vi "Perform Checks.vi"(4 "Owner Path (if applicable)":path, 6 "User VI Owner Status":T1, 8 "error in":errorcluster, 9 "New Filename":string, 10 "Selected Template VI or CTL name (including file extension)":string, 11 "Destination Folder":path) -> (0 "error out":errorcluster, 2 "Validated Filename of VI or CTL to be created (including extension)":string, 3 "Filepath of VI or CTL to be created":path)   [LabVIEW 2022 SP3]
doc: "Performs a few sanity checks in order to ensure that everything is ok before attempting to create a new VI based on these inputs. In other words, performs input validation.\n\nSanity checks:\n1. Destination folder exists\n2. Destination folder does not already contain a file with the same name and extension as is about to be created\n3. Selected Template VI or CTL exists\n4. Owner Library or Class exists (if applicable, meaning if the User VI was owned by a library or class)\n\nReturns a meaningful, informative error if any of the sanity checks failed."
uses:
  Owner Status (enum).ctl
  <vilib>/Utility/error.llb/Trim Whitespace One-Sided.vi
panel:
  # "Development\ncontrols/indicators useful for development and testing, but which are not outputs of the VI"
  # "Input\nInputs to the VI"
  # "Output\nOutputs of the VI"
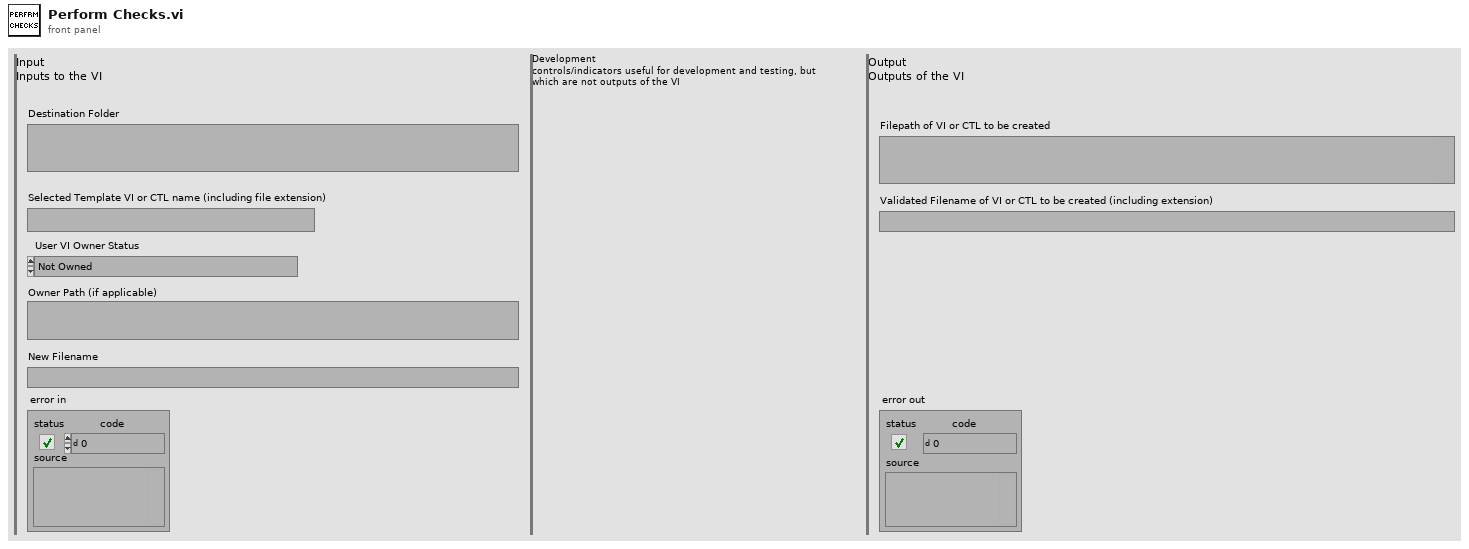
[diagram p1: front panel]
types:
  T1 = typedef "Owner Status (enum).ctl" = enum16{"Not Owned", "Owned by Library (lvlib)", "Owned by Class (lvclass)"}
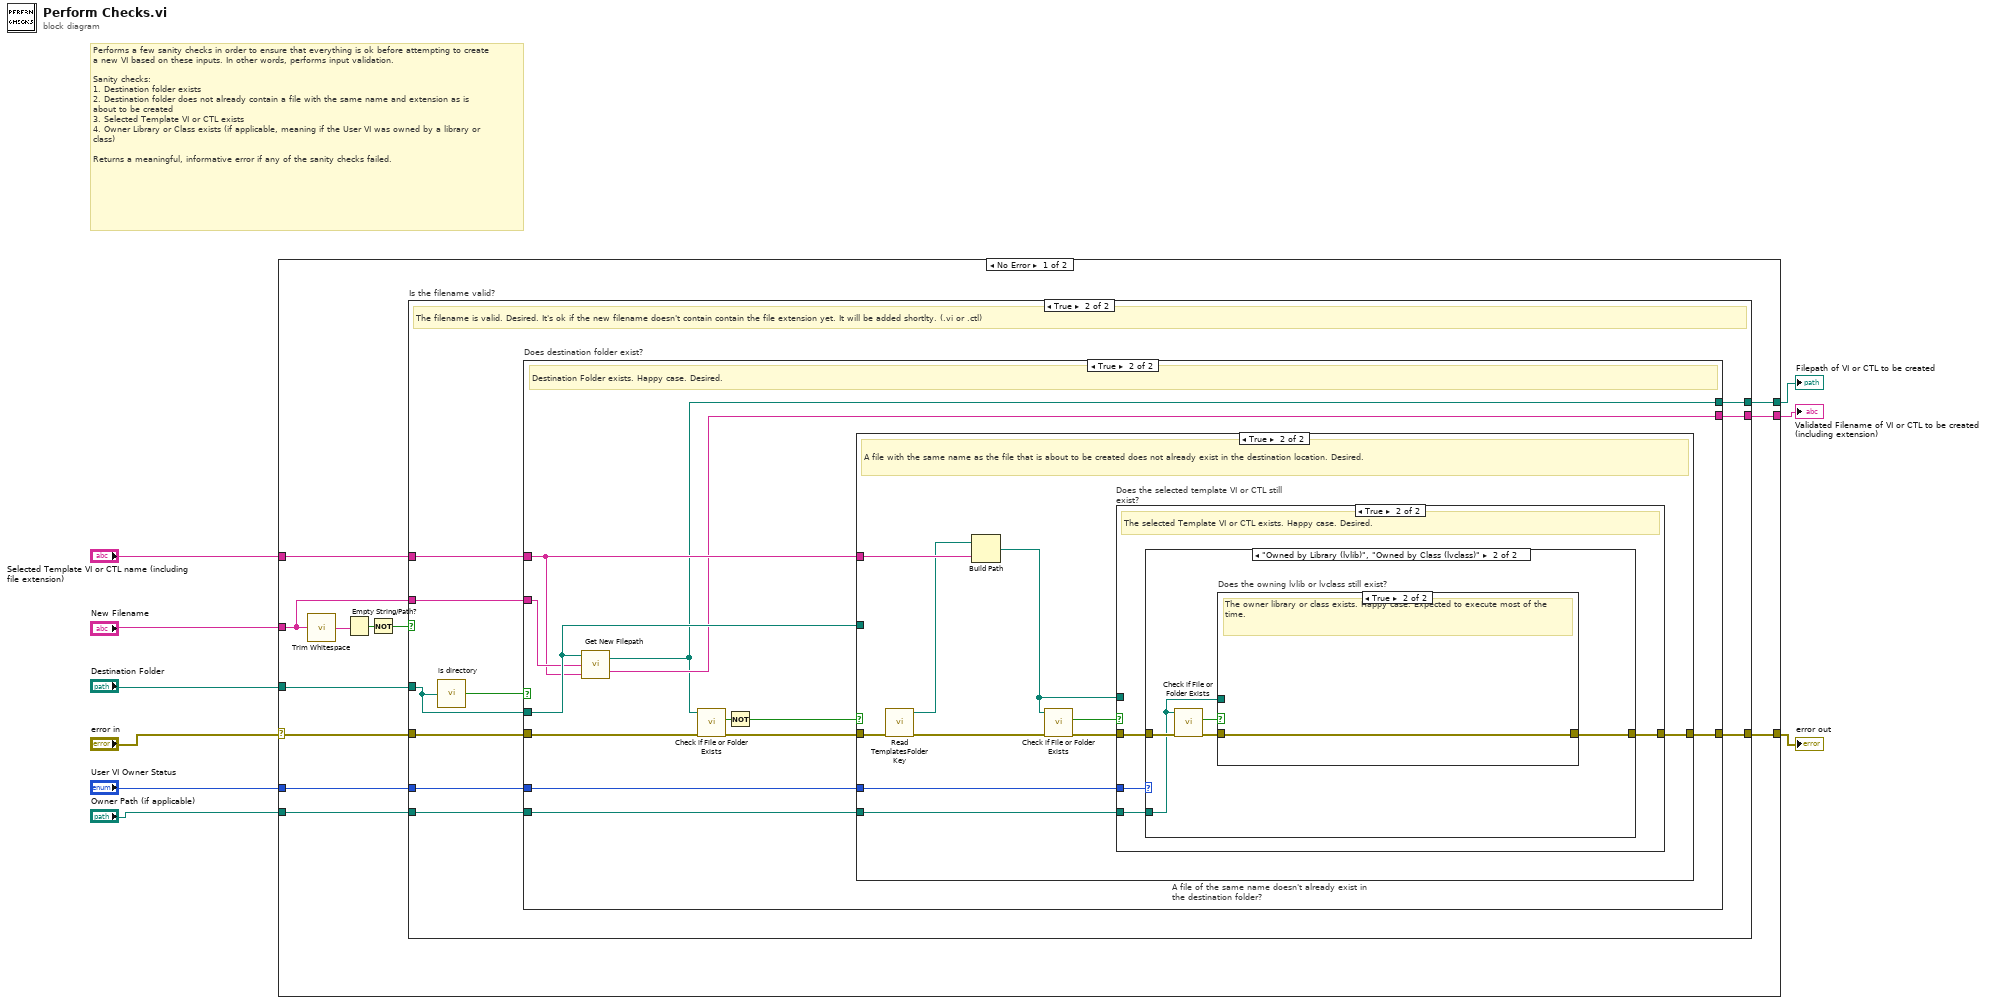
[diagram p0: block diagram]
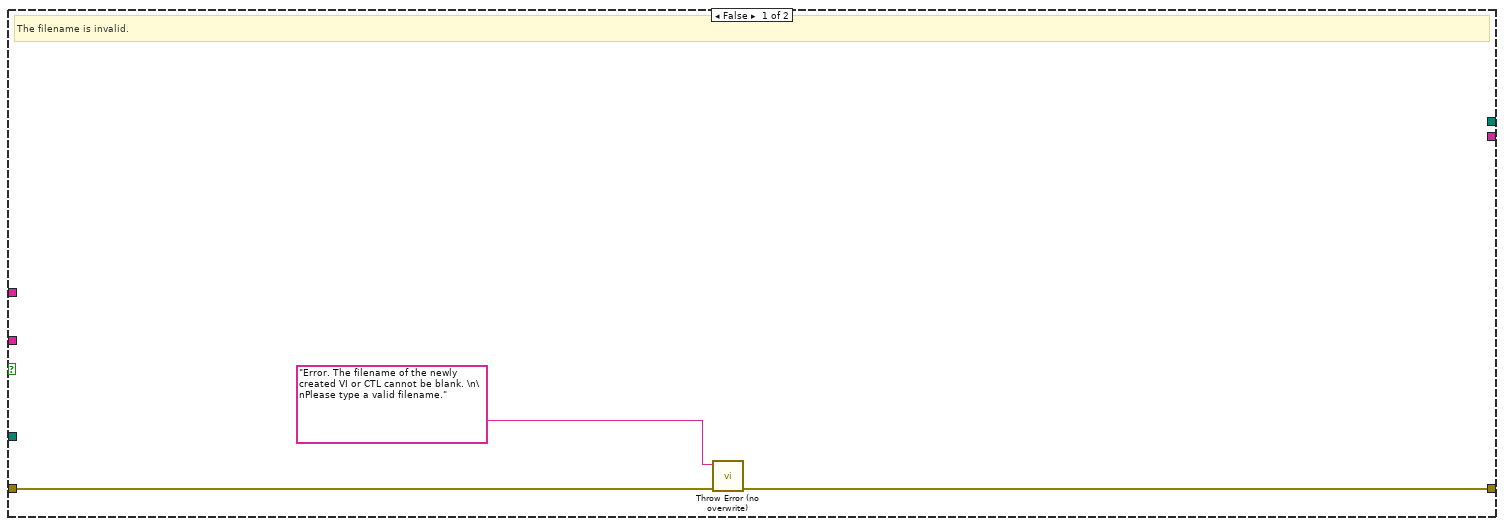
[diagram p2: hidden frame]
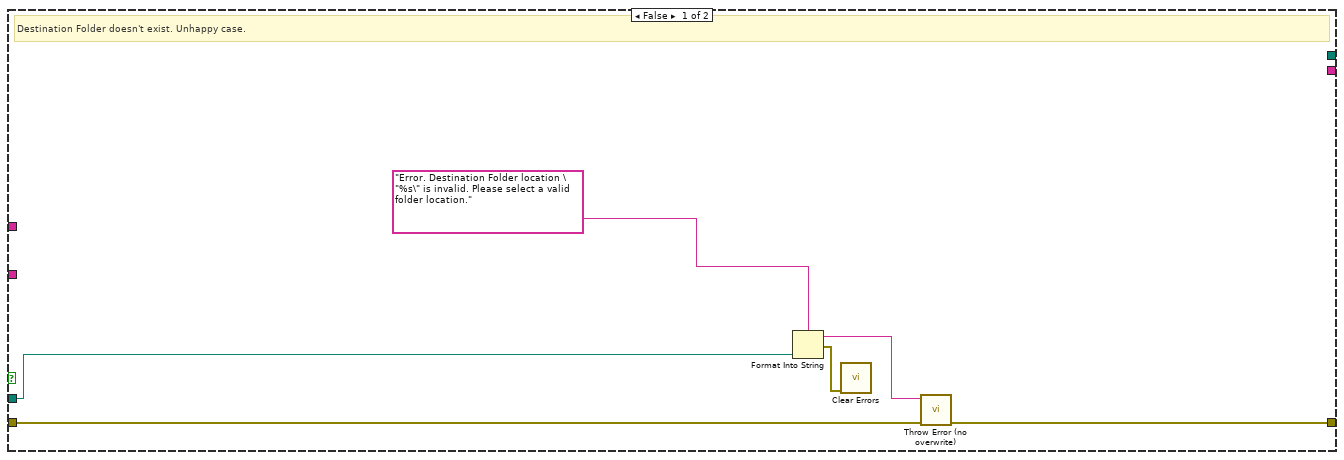
[diagram p3: hidden frame]
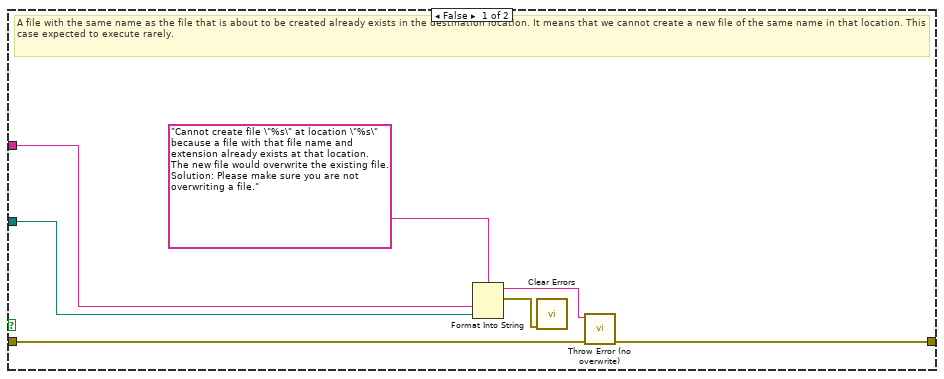
[diagram p4: hidden frame]
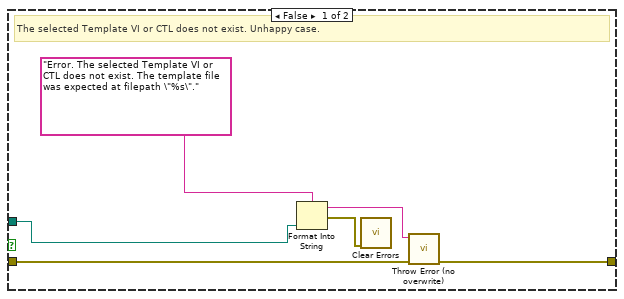
[diagram p5: hidden frame]
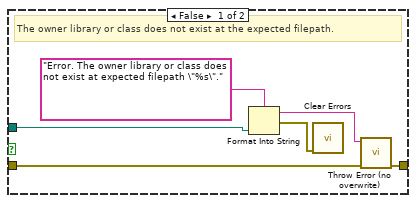
[diagram p7: hidden frame]
diagram:
  # "Performs a few sanity checks in order to ensure that everything is ok before attempting to create a new VI based on these inputs. In other words, performs input validation.\n\nSanity checks:\n1. Destination folder exists\n2. Destination folder does not already contain a file with the same name and extension as is about to be created\n3. Selected Template VI or CTL exists\n4. Owner Library or Class exists (if applicable, meaning if the User VI was owned by a library or class)\n\nReturns a meaningful, informative error if any of the sanity checks failed."
  n1 = case shown="No Error" "error in" {
    selector: "error in" -> [w21 w93]
    tunnel: [w20 w93] -> w8
    tunnel: "Destination Folder" -> [w16 _]
    tunnel: "Selected Template VI or CTL name (including file extension)" -> [w19 _]
    tunnel: "User VI Owner Status" -> [w18 _]
    tunnel: "Owner Path (if applicable)" -> [w17 _]
    tunnel: "New Filename" -> [w12 _]
    tunnel: [w11 _] -> w2
    tunnel: [w10 _] -> w1
    frame No Error {
      n2 = call <vilib>:"Trim Whitespace.vi"("string"=w12) -> ("trimmed string"=w14:string)  [unwired: 1 in]
      n3 = Empty String/Path?(string/path=w14) -> (empty?=w15:bool)
      n4 = Not(x=w15) -> (.not. x?=w13:bool)
      n5 = case "Is the filename valid?" shown="True" w13 {
        tunnel: w21 -> [w23 w34]
        tunnel: [w22 w33] -> w20
        tunnel: w19 -> [_ w32]
        tunnel: w18 -> [_ w31]
        tunnel: w17 -> [_ w30]
        tunnel: w16 -> [_ w29]
        tunnel: w12 -> [_ w27]
        tunnel: [_ w26] -> w11
        tunnel: [_ w25] -> w10
        frame False {
          # "The filename is invalid."
          n6 = call "Throw Error (no overwrite).vi"("error in"=w23, "Error Message"="Error. The filename of the newly created VI or CTL cannot be blank. \n\nPlease type a valid filename.") -> ("error out"=w22:errorcluster)  [unwired: 9 in]
        }
        frame True {
          # "The filename is valid. Desired. It's ok if the new filename doesn't contain contain the file extension yet. It will be added shortlty. (.vi or .ctl)"
          n7 = call "is directory.vi"("Path"=w29) -> ("Does the path point to a directory (a folder)?"=w28:bool)
          n8 = case "Does destination folder exist?" shown="True" w28 {
            tunnel: w34 -> [w40 w48]
            tunnel: [w39 w52] -> w33
            tunnel: w29 -> [w36 w45]
            tunnel: w32 -> [_ w43]
            tunnel: w31 -> [_ w51]
            tunnel: w30 -> [_ w50]
            tunnel: w27 -> [_ w44]
            tunnel: [_ w42] -> w26
            tunnel: [_ w41] -> w25
            frame False {
              # "Destination Folder doesn't exist. Unhappy case."
              n9 = Format Into String(format string="Error. Destination Folder location \"%s\" is invalid. Please select a valid folder location.", w36) -> (resulting string=w35:string, error out=w37:errorcluster)  [unwired: 2 in]
              n10 = call <vilib>:"Clear Errors.vi"("error in (no error)"=w37) -> ()  [unwired: 5 in, 2 out]
              n11 = call "Throw Error (no overwrite).vi"("error in"=w40, "Error Message"=w35) -> ("error out"=w39:errorcluster)  [unwired: 9 in]
            }
            frame True {
              # "Destination Folder exists. Happy case. Desired."
              n12 = call "Get New Filepath.vi"("Selected Template VI or CTL name (including file extension)"=w43, "New Filename"=w44, "Destination Folder"=w45) -> ("Validated Filename of VI or CTL to be created (including extension)"=w42:string, "Filepath of VI or CTL to be created"=w41:path)
              n13 = call <vilib>:"Check if File or Folder Exists.vi"("error in (no error)"=w48, "path"=w41) -> ("error out"=w49:errorcluster, "file or folder exists?"=w47:bool)  [unwired: 7 in, 1 out]
              n14 = Not(x=w47) -> (.not. x?=w46:bool)
              n15 = case "A file of the same name doesn't already exist in the destination folder?" shown="True" w46 {
                tunnel: w43 -> [w54 w69]
                tunnel: w49 -> [w56 w62]
                tunnel: [w55 w65] -> w52
                tunnel: w51 -> [_ w64]
                tunnel: w50 -> [_ w63]
                tunnel: w45 -> [w53 _]
                frame False {
                  # "A file with the same name as the file that is about to be created already exists in the destination location. It means that we cannot create a new file of the same name in that location. This case expected to execute rarely."
                  n16 = Format Into String(format string="Cannot create file \"%s\" at location \"%s\" because a file with that file name and extension already exists at that location. The new file would overwrite the existing file. Solution: Please make sure you are not overwriting a file.", w54, w53) -> (resulting string=w57:string, error out=w58:errorcluster)  [unwired: 2 in]
                  n17 = call <vilib>:"Clear Errors.vi"("error in (no error)"=w58) -> ()  [unwired: 5 in, 2 out]
                  n18 = call "Throw Error (no overwrite).vi"("error in"=w56, "Error Message"=w57) -> ("error out"=w55:errorcluster)  [unwired: 9 in]
                }
                frame True {
                  # "A file with the same name as the file that is about to be created does not already exist in the destination location. Desired."
                  n19 = call "Read TemplatesFolder Key.vi"("Error In"=w62) -> ("Error Out"=w61:errorcluster, "Templates Folder Path"=w60:path)  [unwired: 9 in]
                  n20 = Build Path(base path=w60, name or relative path=w69) -> (appended path=w66:path)
                  n21 = call <vilib>:"Check if File or Folder Exists.vi"("error in (no error)"=w61, "path"=w66) -> ("error out"=w68:errorcluster, "file or folder exists?"=w67:bool)  [unwired: 7 in, 1 out]
                  n22 = case "Does the selected template VI or CTL still exist?" shown="True" w67 {
                    tunnel: w68 -> [w75 w79]
                    tunnel: w66 -> [w71 _]
                    tunnel: [w70 w78] -> w65
                    tunnel: w64 -> [_ w77]
                    tunnel: w63 -> [_ w76]
                    frame False {
                      # "The selected Template VI or CTL does not exist. Unhappy case."
                      n23 = Format Into String(format string="Error. The selected Template VI or CTL does not exist. The template file was expected at filepath \"%s\".", w71) -> (resulting string=w72:string, error out=w73:errorcluster)  [unwired: 2 in]
                      n24 = call <vilib>:"Clear Errors.vi"("error in (no error)"=w73) -> ()  [unwired: 5 in, 2 out]
                      n25 = call "Throw Error (no overwrite).vi"("error in"=w75, "Error Message"=w72) -> ("error out"=w70:errorcluster)  [unwired: 9 in]
                    }
                    frame True {
                      # "The selected Template VI or CTL exists. Happy case. Desired."
                      n26 = case shown="\"Owned by Library (lvlib)\", \"Owned by Class (lvclass)\"" w77 {
                        tunnel: w79 -> [w80 w85]
                        tunnel: [w80 w83] -> w78
                        tunnel: w76 -> [_ w81]
                        frame "Not Owned" {
                        }
                        frame "Owned by Library (lvlib)", "Owned by Class (lvclass)" {
                          n27 = call <vilib>:"Check if File or Folder Exists.vi"("error in (no error)"=w85, "path"=w81) -> ("error out"=w84:errorcluster, "file or folder exists?"=w82:bool)  [unwired: 7 in, 1 out]
                          n28 = case "Does the owning lvlib or lvclass still exist?" shown="True" w82 {
                            tunnel: w84 -> [w88 w92]
                            tunnel: [w87 w92] -> w83
                            tunnel: w81 -> [w86 _]
                            frame False {
                              # "The owner library or class does not exist at the expected filepath."
                              n29 = Format Into String(format string="Error. The owner library or class does not exist at expected filepath \"%s\".", w86) -> (resulting string=w89:string, error out=w90:errorcluster)  [unwired: 2 in]
                              n30 = call <vilib>:"Clear Errors.vi"("error in (no error)"=w90) -> ()  [unwired: 5 in, 2 out]
                              n31 = call "Throw Error (no overwrite).vi"("error in"=w88, "Error Message"=w89) -> ("error out"=w87:errorcluster)  [unwired: 9 in]
                            }
                            frame True {
                              # "The owner library or class exists. Happy case. Expected to execute most of the time."
                            }
                          }
                        }
                      }
                    }
                  }
                }
              }
            }
          }
        }
      }
    }
    frame Error {
    }
  }
  "error out" <- w8
  "Validated Filename of VI or CTL to be created (including extension)" <- w2
  "Filepath of VI or CTL to be created" <- w1
